vi "ctx get max sample delay seconds.vi"(10 "dest":u16, 11 "context":u32) -> (1 "function return":i32, 2 "dest out":u16, 3 "context out":u32)   [LabVIEW 2019, in "apdm.lvlib"]
doc: "APDM_EXPORT int apdm_ctx_get_max_sample_delay_seconds(apdm_ctx_t context, uint16_t *dest);"
uses:
  apdm.lvlib
  Lee Lab/CP FES Walking 2018/Code/Working/LabVIEW/apdm.dll
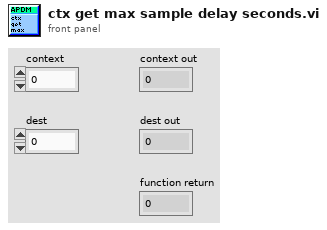
[diagram p1: front panel]
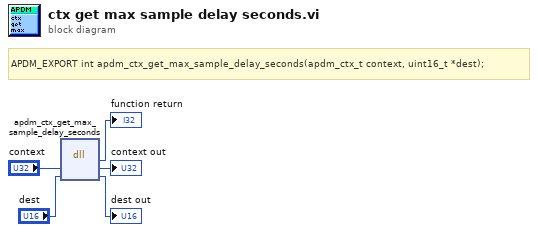
[diagram p0: block diagram]
diagram:
  # "APDM_EXPORT int apdm_ctx_get_max_sample_delay_seconds(apdm_ctx_t context, uint16_t *dest);"
  n1 = dll-call lib="C:/Users/jfalesi/Dropbox/Lee Lab/CP FES Walking 2018/Code/Working/LabVIEW/apdm.*" fn="apdm_ctx_get_max_sample_delay_seconds"("context"="context", "dest"="dest") -> (→"function return":i32, "context"=→"context out":u32, "dest"=→"dest out":u16)  [unwired: 3 in, 2 out]
